vi "FPS Counter.vi"() -> (3 "Numeric":dbl)   [LabVIEW 2017]
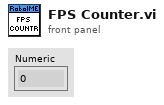
[diagram p1: front panel]
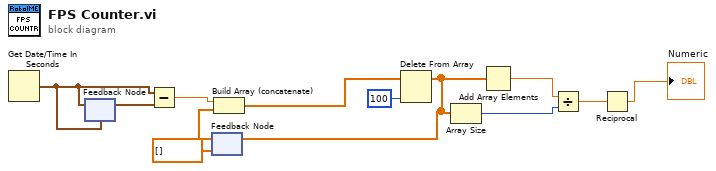
[diagram p0: block diagram]
diagram:
  n1 = Get Date/Time In Seconds() -> (seconds since 1Jan1904=w1:timestamp)
  n2 = feedback #1(w1) -> (w2:timestamp)
  n3 = feedback-in #1(w1) -> ()
  n4 = Subtract(x=w1, y=w2) -> (x-y=w3:dbl)
  n5 = feedback #2(dbl[] []) -> (w4:dbl[])
  n6 = Build Array (concatenate)(w3, w4) -> (w6:dbl[])
  n7 = Delete From Array(array=w6, index=100) -> (array with subset deleted=w10:dbl[])  [unwired: 1 in, 1 out]
  n8 = feedback-in #2(w10) -> ()
  n9 = Array Size(array=w10) -> (size(s)=w9:i32)
  n10 = Add Array Elements(numeric array=w10) -> (sum=w8:dbl)
  n11 = Divide(x=w8, y=w9) -> (x/y=w11:dbl)
  n12 = Reciprocal(x=w11) -> (1/x=→"Numeric":dbl)
